vi "verify camera op mode error.vi"(8 "error in (no error)":errorcluster, 11 "Channel in":refnum<class "Channel.lvclass">) -> (0 "error out":errorcluster, 2 "logical OR":bool, 3 "Channel out":refnum<class "Channel.lvclass">)   [LabVIEW 2018, in "Channel.lvclass"]
uses:
  Channel.lvclass
  Channel.lvclass/Channel.ctl
  Simulated_CCD_Camera/Simulated Camera.lvclass/Simulated Camera.ctl
  Simulated_CCD_Camera/Simulated Camera.lvclass
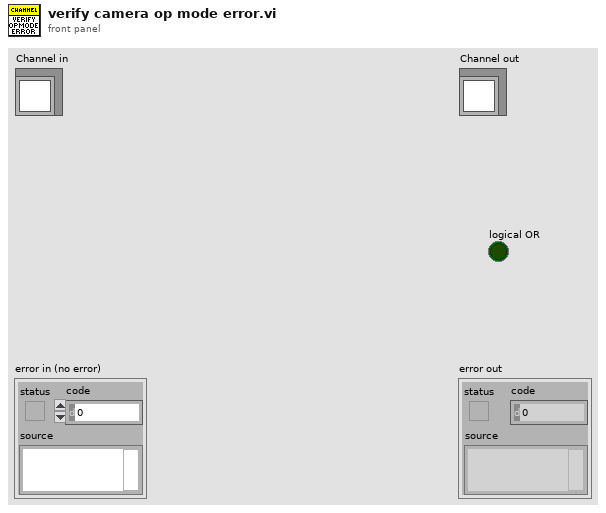
[diagram p1: front panel]
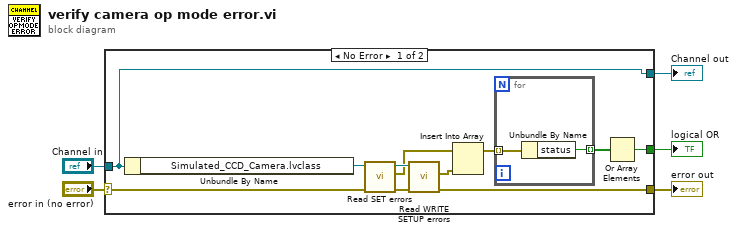
[diagram p0: block diagram]
diagram:
  n1 = case shown="No Error" "error in (no error)" {
    selector: "error in (no error)" -> [w8 w20]
    tunnel: [w7 w20] -> w4
    tunnel: [w10 w19] -> w2
    tunnel: "Channel in" -> [w10 w19]
    tunnel: [w6 _] -> w1
    frame No Error {
      n2 = Unbundle By Name(w10) -> ("Simulated_CCD_Camera.lvclass"=w9:refnum<class "Simulated Camera.lvclass">)
      n3 = call-dynamic "Read SET errors.vi"("error in (no error)"=w8, "Simulated Camera in"=w9) -> ("error out"=w15:errorcluster, "SET errors"=w13:errorcluster[], "Simulated Camera out"=w14:refnum<class "Simulated Camera.lvclass">)  [unwired: 7 in]
      n4 = call "Read WRITE SETUP errors.vi"("error in (no error)"=w15, "Simulated_CCD_Camera in"=w14) -> ("error out"=w7:errorcluster, "WRITE SETUP errors"=w12:errorcluster[])  [unwired: 7 in, 1 out]
      n5 = Insert Into Array(array=w13, new element=w12) -> (w11:errorcluster[])  [unwired: 1 in]
      n6 = for {
        tunnel: [w18] -> w16 mode=indexing
        tunnel: w11 -> [w17] mode=indexing
        n7 = Unbundle By Name(w17) -> ("status"=w18:bool)
      }
      n8 = Or Array Elements(Boolean array=w16) -> (logical OR=w6:bool)
    }
    frame Error {
    }
  }
  "error out" <- w4
  "Channel out" <- w2
  "logical OR" <- w1
